vi "__fpgaChirpData.vi"(9 "sample_rate":dbl, 10 "icfft":i32) -> (3 "ReturnValue":i32, 11 "cx_ChirpDataArray":csg[](array[numeric]))   [LabVIEW 2015]
uses:
  SETI_LV/FGV/SETI_LV_FGV.ctl
  SETI_LV/SETI_LV.lvlib
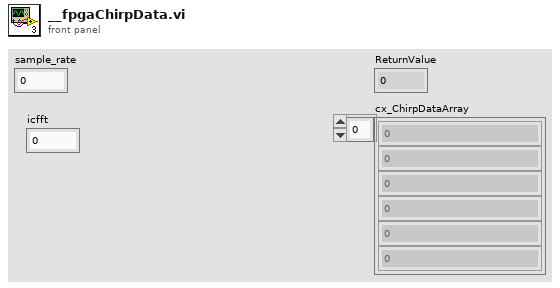
[diagram p1: front panel]
types:
  T1 = typedef "SETI_LV.lvlib/SETI_LV_FGV.ctl" = enum16{"Get", "Set", "Chirp(icfft)"}
  T2 = typedef "SETI_LV.lvlib/ChirpFFT Pairs.ctl" = cluster{"Chirp/Fft Pair 1 - Chirp Rate":dbl, "Chirp/Fft Pair 1 - Chirp Rate Ind":i32, "Chirp/Fft Pair 1 - Fft Length":i32, "Chirp/Fft Pair 1 - Pulse Find":i32, "Chirp/Fft Pair 1 - Gauss Fit":i32}
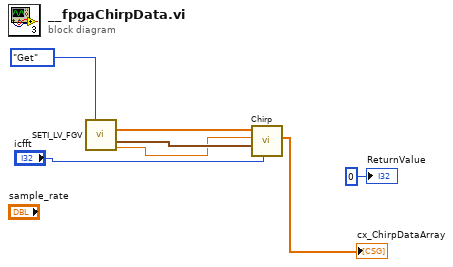
[diagram p0: block diagram]
diagram:
  n1 = call "SETI_LV_FGV.vi"("Command"=SETI_LV_FGV."Get") -> ("DataIn out"=w5:csg[], "Chirp FFT Pairs out"=w4:T2[], "subband_sample_rate out"=w3:dbl)  [unwired: 10 in, 2 out]
  n2 = call "Chirp.vi"("icfft"="icfft", "Chirp FFT Pairs"=w4, "Sub-band Sample Rate"=w3, "binWorkUnitDataPoints.bin (DataIn) in"=w5) -> ("binWorkUnitDataPoints.bin (DataIn) out"=→"cx_ChirpDataArray":csg[])  [unwired: 1 in, 6 out]
  "ReturnValue" <- 0 ("ReturnValue")
